vi "Movimiento de motores.vi"(8 "error in (no error)":errorcluster, 9 "Tipo de control":T2, 11 "Parametros de control":T1={"Setpoint"=0.0, "PV"=0.0, "Frecuencia PWM"=0.0, "Ciclo de trabajo PWM"=2.5e-06, "V. histeresis (grados)"=0.0, "Ganacias PID"={"proportional gain (Kc)"=1.0, "integral time (Ti, min)"=0.01, "derivative time (Td, min)"=0.0}, "Ref array"=[]} {"Ciclo de trabajo PWM" min=2.5e-06 max=1.0 step=0.1}) -> (0 "error out":errorcluster, 1 "DOs":bool[](array[boolean]), 2 "duty cycle":dbl=0.5 format="%_6g", 3 "frequency":dbl=1.0 format="%_6g")   [LabVIEW 2018]
uses:
  <vilib>/addons/control/pid/NI_PID_pid.lvlib
  <vilib>/addons/control/pid/pid.llb/PID Percentage to EGU (DBL).vi
  <vilib>/addons/control/pid/_prctrl compat.llb/PID (Compatibility).vi
  <vilib>/addons/control/pid/NI_PID__prctrl compat.lvlib
  typedef/Selector control.ctl
  typedef/Parametros control.ctl
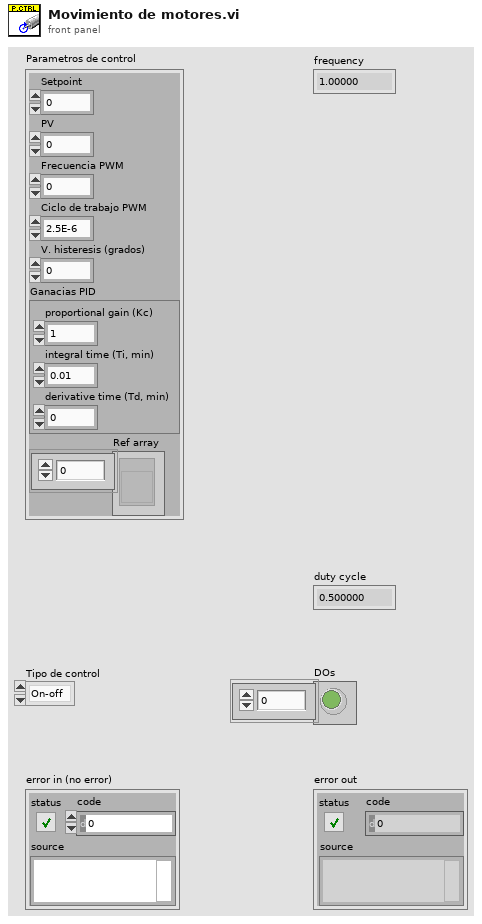
[diagram p1: front panel]
types:
  T1 = typedef "Parametros control.ctl" = cluster{"Setpoint":dbl, "PV":dbl, "Frecuencia PWM":dbl, "Ciclo de trabajo PWM":dbl, "V. histeresis (grados)":dbl, "Ganacias PID":cluster{"proportional gain (Kc)":dbl, "integral time (Ti, min)":dbl, "derivative time (Td, min)":dbl}, "Ref array":refnum<vi>[]}
  T2 = typedef "Selector control.ctl" = enum16{"On-off", "On-off hist.", "PID"}
  T3 = cluster{"sp low":dbl, "sp high":dbl, "out low":dbl, "out high":dbl, "hold (F)":bool, "auto (T)":bool, "pro. band (F)":bool, "reverse acting (T)":bool, "beta":dbl, "linearity":dbl, "dt (s)":dbl}
  T4 = cluster{"proportional gain (Kc)":dbl, "integral time (Ti, min)":dbl, "derivative time (Td, min)":dbl}
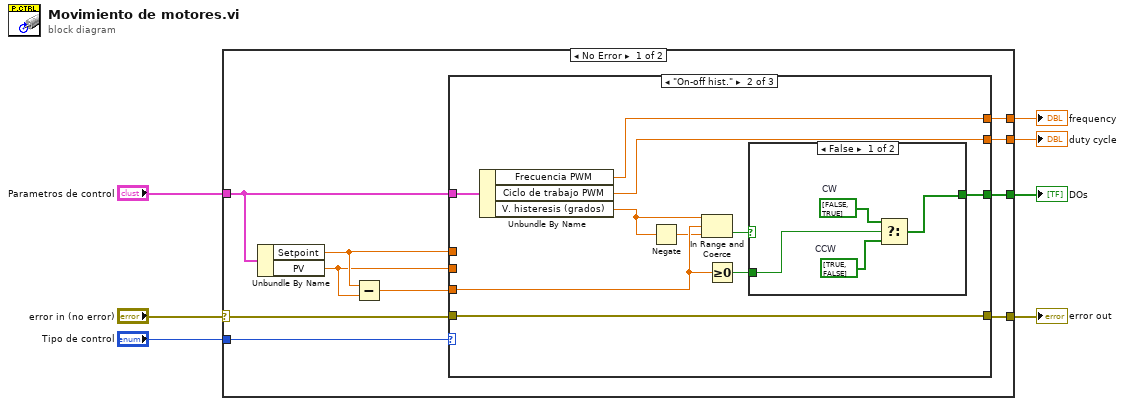
[diagram p0: block diagram]
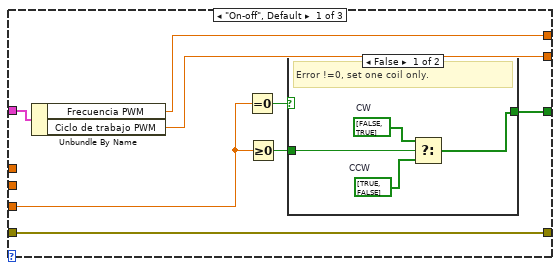
[diagram p2: hidden frame]
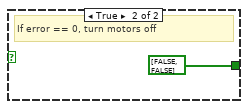
[diagram p3: hidden frame]
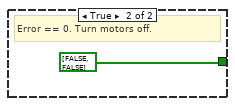
[diagram p4: hidden frame]
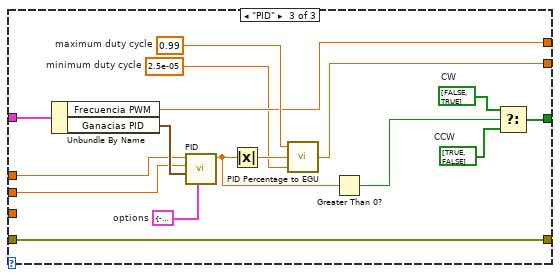
[diagram p5: hidden frame]
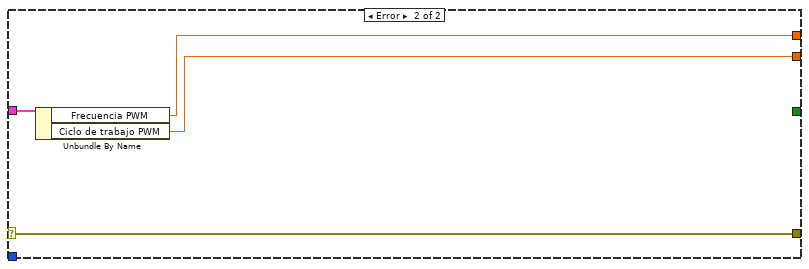
[diagram p6: hidden frame]
diagram:
  n1 = case shown="No Error" "error in (no error)" {
    selector: "error in (no error)" -> [w17 w65]
    tunnel: [w16 w65] -> w6
    tunnel: "Parametros de control" -> [w14 w64]
    tunnel: "Tipo de control" -> [w15 _]
    tunnel: [w10 w63] -> w3
    tunnel: [w9 _] -> w2
    tunnel: [w8 w62] -> w1
    frame No Error {
      n2 = Unbundle By Name(w14) -> ("Setpoint"=w12:dbl, "PV"=w11:dbl)
      n3 = Subtract(x=w12, y=w11) -> (x-y=w13:dbl)
      n4 = case shown="\"On-off hist.\"" w15 {
        tunnel: w13 -> [w25 w38 _]
        tunnel: w14 -> [w24 w40 w61]
        tunnel: w17 -> [w23 w39 w59]
        tunnel: [w23 w39 w59] -> w16
        tunnel: w12 -> [_ _ w55]
        tunnel: w11 -> [_ _ w54]
        tunnel: [w22 w35 w52] -> w10
        tunnel: [w20 w32 w46] -> w9
        tunnel: [w19 w34 w51] -> w8
        frame "On-off", Default {
          n5 = Unbundle By Name(w24) -> ("Frecuencia PWM"=w22:dbl, "Ciclo de trabajo PWM"=w19:dbl)
          n6 = Equal To 0?(x=w25) -> (x = 0?=w21:bool)
          n7 = Greater Or Equal To 0?(x=w25) -> (x >= 0?=w18:bool)
          n8 = case shown="False" w21 {
            tunnel: [w26 bool[] [FALSE, FALSE] ("DOs")] -> w20
            tunnel: w18 -> [w29 _]
            frame False {
              w27 = bool[] [TRUE, FALSE]  # CCW
              w28 = bool[] [FALSE, TRUE]  # CW
              # "Error !=0, set one coil only."
              n9 = Select(t=w28, s=w29, f=w27) -> (s? t:f=w26:bool[])
            }
            frame True {
              # "If error == 0, turn motors off"
            }
          }
        }
        frame "On-off hist." {
          n10 = Unbundle By Name(w40) -> ("Frecuencia PWM"=w35:dbl, "Ciclo de trabajo PWM"=w34:dbl, "V. histeresis (grados)"=w36:dbl)
          n11 = Negate(x=w36) -> (-x=w37:dbl)
          n12 = In Range and Coerce(upper limit=w36, x=w38, lower limit=w37) -> (In Range?=w33:bool)  [unwired: 1 out]
          n13 = Greater Or Equal To 0?(x=w38) -> (x >= 0?=w31:bool)
          n14 = case shown="False" w33 {
            tunnel: [w41 bool[] [FALSE, FALSE] ("DOs")] -> w32
            tunnel: w31 -> [w42 _]
            frame False {
              w43 = bool[] [TRUE, FALSE]  # CCW
              w44 = bool[] [FALSE, TRUE]  # CW
              n15 = Select(t=w44, s=w42, f=w43) -> (s? t:f=w41:bool[])
            }
            frame True {
              # "Error == 0. Turn motors off."
            }
          }
        }
        frame "PID" {
          w48 = bool[] [TRUE, FALSE]  # CCW
          w49 = bool[] [FALSE, TRUE]  # CW
          w50 = 2.5e-05  # minimum duty cycle
          w53 = T3 {"sp low"=-180.0, "sp high"=180.0, "out low"=-170.0, "out high"=170.0, "hold (F)"=FALSE, "auto (T)"=TRUE, "pro. band (F)"=FALSE, "reverse acting (T)"=TRUE, "beta"=1.0, "linearity"=1.0, "dt (s)"=-1.0}  # options
          w58 = 0.99  # maximum duty cycle
          n16 = Unbundle By Name(w61) -> ("Frecuencia PWM"=w52:dbl, "Ganacias PID"=w60:T4)
          n17 = call-poly <vilib>:"PID.vi"("options"=w53, "PID parameters"=w60, "process variable"=w54, "setpoint"=w55) -> ("output"=w57:dbl)  [unwired: 7 in]
          n18 = Absolute Value(x=w57) -> (abs(x)=w56:dbl)
          n19 = call-poly <vilib>:"PID Percentage to EGU.vi"("minimum (EGU)"=w50, "% span"=w56, "maximum (EGU)"=w58) -> ("output (EGU)"=w51:dbl)  [unwired: 1 in]
          n20 = Greater Than 0?(x=w57) -> (x > 0?=w47:bool)
          n21 = Select(t=w49, s=w47, f=w48) -> (s? t:f=w46:bool[])
        }
      }
    }
    frame Error {
      n22 = Unbundle By Name(w64) -> ("Frecuencia PWM"=w63:dbl, "Ciclo de trabajo PWM"=w62:dbl)
    }
  }
  "error out" <- w6
  "frequency" <- w3
  "duty cycle" <- w1
  "DOs" <- w2
